vi "Check Safety.vi"(8 "error in (no error)":errorcluster, 11 "VacuumLine in":refnum<class "VacuumLine.lvclass">) -> (0 "error out":errorcluster, 3 "VacuumLine out":refnum<class "VacuumLine.lvclass">, 5 "Error":bool)   [LabVIEW 2016, in "Hardware.lvlib" / "VacuumLine.lvlib" / "VacuumLine.lvclass"]
uses:
  <userlib>/Common Components/Hardware/Abstract System/VacuumLine/VacuumLine/VacuumLine.lvclass
  <userlib>/Common Components/Hardware/Abstract System/VacuumLine/VacuumLine/VacuumLine.lvclass/VacuumLine.ctl
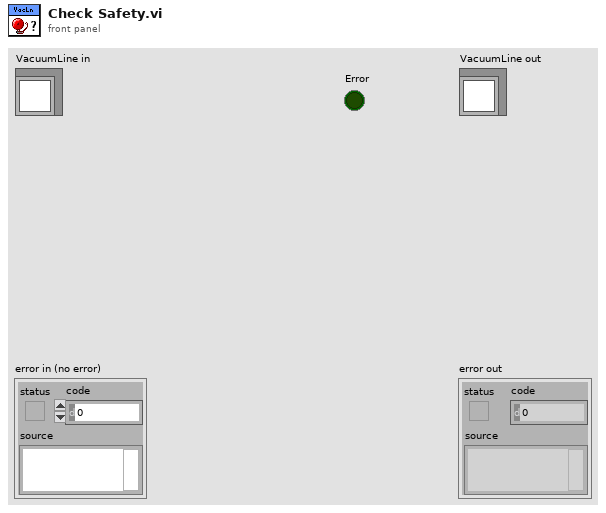
[diagram p1: front panel]
types:
  T1 = cluster{"valve":bool, "optical switch -":bool, "optical switch +":bool, "Valve Closed Status Alert":bool}[]
  T2 = typedef "Hardware.lvlib/VacuumLine.lvlib/VacuumLine.lvclass/Valve Complex.ctl" = cluster{"LogicIO Module":string, "Valve Open":T3, "Optical Switch -":T3, "Optical Switch +":T3, "Valve Closed Status Alert":cluster{"Pin#":u8, "Option":enum16{"Not Used", "Normally Closed"}}}
  T3 = typedef "Hardware.lvlib/VacuumLine.lvlib/VacuumLine.lvclass/Logic Cluster.ctl" = cluster{"Pin#":u8, "Location":dbl, "Tolerance":dbl}
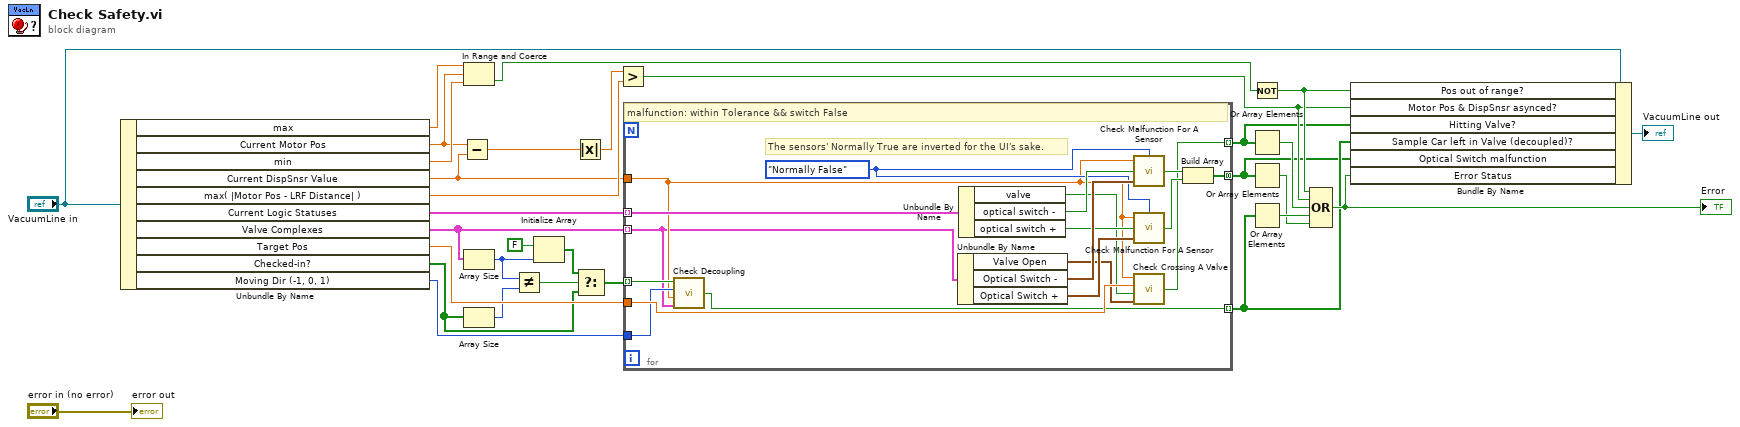
[diagram p0: block diagram]
diagram:
  n1 = Unbundle By Name("VacuumLine in") -> ("max"=w29:dbl, "Current Motor Pos"=w26:dbl, "min"=w28:dbl, "Current DispSnsr Value"=w8:dbl, "max( |Motor Pos - LRF Distance| )"=w23:dbl, "Current Logic Statuses"=w22:T1, "Valve Complexes"=w10:T2[], "Target Pos"=w21:dbl, "Checked-in?"=w11:bool[], "Moving Dir (-1, 0, 1)"=w20:i32)
  n2 = Subtract(x=w26, y=w8) -> (x-y=w25:dbl)
  n3 = In Range and Coerce(upper limit=w29, x=w26, lower limit=w28) -> (In Range?=w27:bool)  [unwired: 1 out]
  n4 = Array Size(array=w10) -> (size(s)=w13:i32)
  n5 = Array Size(array=w11) -> (size(s)=w16:i32)
  n6 = Not Equal?(x=w13, y=w16) -> (x != y?=w15:bool)
  n7 = Initialize Array(FALSE, w13) -> (w12:bool[])
  n8 = Absolute Value(x=w25) -> (abs(x)=w24:dbl)
  n9 = Select(t=w12, s=w15, f=w11) -> (s? t:f=w9:bool[])
  n10 = Greater?(x=w24, y=w23) -> (0:w4:bool)
  n11 = for {
    tunnel: w10 -> [w33] mode=indexing
    tunnel: w8 -> [w34]
    tunnel: w22 -> [w49] mode=indexing
    tunnel: [w41] -> w1 mode=concatenating
    tunnel: w21 -> [w40]
    tunnel: [w37] -> w3 mode=indexing
    tunnel: w9 -> [w36] mode=indexing
    tunnel: w20 -> [w35]
    tunnel: [w32] -> w2 mode=indexing
    w44 = enum16{"Normally True", "Normally False"}."Normally False" ("Mode")
    # "The sensors' Normally True are inverted for the UI's sake."
    # "malfunction: within Tolerance && switch False"
    n12 = call <userlib>:"Check Decoupling.vi"("Valve package"=w33, "Current Pos"=w34, "Moving Dir (-1, 0, 1)"=w35, "Checked-in?"=w36) -> ("Sample Car left in Valve (decoupled)?"=w32:bool)
    n13 = Unbundle By Name(w33) -> ("Valve Open"=w38:T3, "Optical Switch -"=w47:T3, "Optical Switch +"=w45:T3)
    n14 = Unbundle By Name(w49) -> ("valve"=w39:bool, "optical switch -"=w48:bool, "optical switch +"=w46:bool)
    n15 = call <userlib>:"Check Malfunction For A Sensor.vi"("Mode"=w44, "Logic Cluster"=w47, "Logic Status"=w48, "Current Pos"=w34) -> ("Malfunction?"=w43:bool)
    n16 = call <userlib>:"Check Malfunction For A Sensor.vi"("Mode"=w44, "Logic Cluster"=w45, "Logic Status"=w46, "Current Pos"=w34) -> ("Malfunction?"=w42:bool)
    n17 = call <userlib>:"Check Crossing A Valve.vi"("Logic Cluster"=w38, "Valve Open?"=w39, "Target Pos"=w40, "Current Pos"=w34) -> ("Crossing Valve Error"=w37:bool)
    n18 = Build Array(w43, w42) -> (w41:bool[])
  }
  n19 = Not(x=w27) -> (.not. x?=w5:bool)
  n20 = Or Array Elements(Boolean array=w3) -> (logical OR=w19:bool)
  n21 = Or Array Elements(Boolean array=w1) -> (logical OR=w17:bool)
  n22 = Or Array Elements(Boolean array=w2) -> (logical OR=w18:bool)
  n23 = Compound Arithmetic op=OR(w5, w4, w19, w18, w17) -> (w6:bool)
  "Error" <- w6
  n24 = Bundle By Name(cluster="VacuumLine in", "Pos out of range?"=w5, "Motor Pos & DispSnsr asynced?"=w4, "Hitting Valve?"=w3, "Sample Car left in Valve (decoupled)?"=w2, "Optical Switch malfunction"=w1, "Error Status"=w6) -> (→"VacuumLine out":refnum<class "VacuumLine.lvclass">)
  "error out" <- "error in (no error)"
